vi "Configure Load Trigger Binning.vi"(0 "VISA resource name":refnum<visa-resource-name>, 1 "Start Delay (0)":dbl, 2 "Limit X Low (1)":i32=1, 5 "Templates (0: GradeBinning)":i32(ring) items=["GradeBinning", "SortBinning"], 7 "Components (1)":i32=1, 9 "Start In Line (5)":i32=5, 11 "error in (no error)":errorcluster, 12 "End Delay (0)":dbl, 13 "Limit X High (1)":i32=1) -> (4 "VISA resource name out":refnum<visa-resource-name>, 15 "error out":errorcluster)   [LabVIEW 2020, in "Keithley DMM6500 DAQ6500 Series.lvlib"]
doc: "Load the bining trigger with the argument"
uses:
  <instrlib>/Keithley DMM6500 DAQ6500 Series/Keithley DMM6500 DAQ6500 Series.lvlib
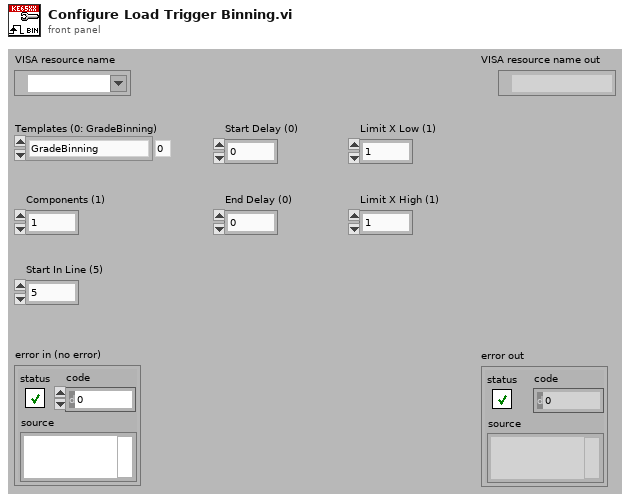
[diagram p1: front panel]
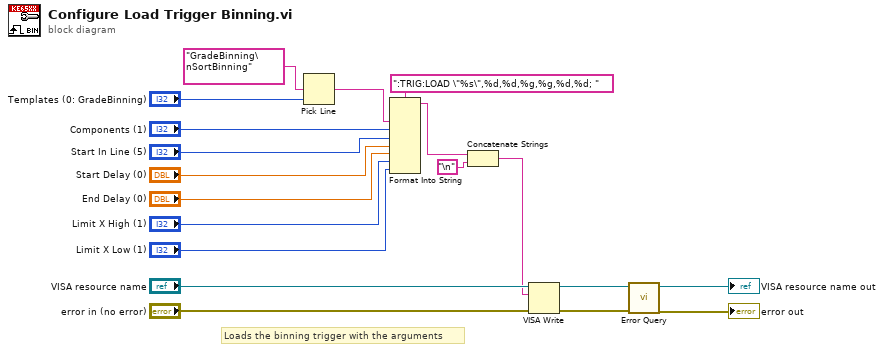
[diagram p0: block diagram]
diagram:
  # "Loads the binning trigger with the arguments"
  n1 = Pick Line(multi-line string="GradeBinning\nSortBinning", line index="Templates (0: GradeBinning)") -> (output string=w12:string)  [unwired: 1 in]
  n2 = Format Into String(format string=":TRIG:LOAD \"%s\",%d,%d,%g,%g,%d,%d; ", w12, "Components (1)", "Start In Line (5)", "Start Delay (0)", "End Delay (0)", "Limit X High (1)", "Limit X Low (1)") -> (resulting string=w8:string)  [unwired: 2 in, 1 out]
  n3 = Concatenate Strings(w8, "\n") -> (w9:string)
  n4 = VISA Write(VISA resource name="VISA resource name", write buffer=w9, error in (no error)="error in (no error)") -> (VISA resource name out=w16:refnum<visa-resource-name>, error out=w15:errorcluster)  [unwired: 1 out]
  n5 = call <instrlib>:"Error Query.vi"("error in (no error)"=w15, "VISA resource name"=w16) -> ("error out"=→"error out":errorcluster, "VISA resource name out"=→"VISA resource name out":refnum<visa-resource-name>)  [unwired: 6 in, 2 out]
